vi "KLN_Query.vi"(0 "System no.":i32=1 min=1 max=4 step=1, 2 "Names to query":string[](array[string]), 5 "error in":errorcluster) -> (14 "Response":string, 19 "error out":errorcluster)   [LabVIEW 2020]
doc: "Returns coordinate system chains. A chain consists of minimum two linked coordinate systems. In case of a cyclic definition the reported chain ends with the cyclic coordinate system.\n\nC-887, F-206, M-8X0: Only for GCS syntax version = GCS 2.0 or higher (Check with CSV?.vi. If CSV?.vi is not supported, syntax version is GCS 1.0)."
panel:
  # "Returns coordinate system chains. A chain consists of minimum two linked coordinate systems."
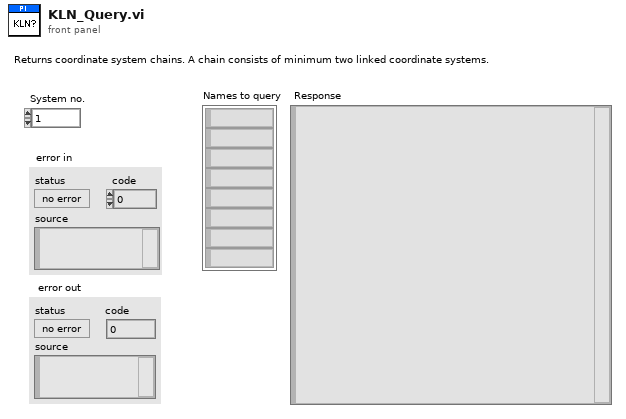
[diagram p1: front panel]
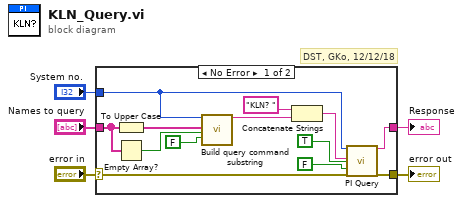
[diagram p0: block diagram]
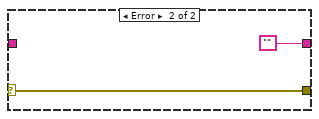
[diagram p2: hidden frame]
diagram:
  # "DST, GKo, 12/12/18"
  n1 = case shown="No Error" "error in" {
    selector: "error in" -> [w8 w19]
    tunnel: "Names to query" -> [w7 _]
    tunnel: [w9 w19] -> w4
    tunnel: "System no." -> [w13 _]
    tunnel: [w10 "" ("String read")] -> w2
    frame No Error {
      n2 = To Upper Case(1:w7) -> (0:w15:string[])
      n3 = Empty Array?(array=w7) -> (empty?=w6:bool)
      n4 = call "Build query command substring.vi"("System no."=w13, "Axes to query in"=w15, "Query\nAll axes?"=w6, "For all axes: use\nAxis identifier?"=FALSE ("For all axes: use\nAxis identifier?")) -> ("Command substring"=w14:string)  [unwired: 2 in, 13 out]
      n5 = Concatenate Strings("KLN? ", w14) -> (w16:string)
      n6 = call "PI Query.vi"("System no."=w13, "String to send"=w16, "Attach termination char.?"=TRUE ("Attach Linefeed?"), "Strip spaces?"=FALSE, "error in"=w8) -> ("String read"=w10:string, "error out"=w9:errorcluster)  [unwired: 2 in, 11 out]
    }
    frame Error {
    }
  }
  "error out" <- w4
  "Response" <- w2
